vi "Starter Kit FPGA Main.vi"() -> ()   [LabVIEW 2017, in "NI_Robotics_Starter Kit 1.0 FPGA.lvlib"]
doc: "This VI implements the low level control of the motors and sensor for the Starter Kit robot."
uses:
  <vilib>/robotics/Starter Kit/1.0/FPGA Source/NI_Robotics_Starter Kit 1.0 FPGA.lvlib
  <vilib>/Platform/TimedLoop/XDataNode/XDataNode.xnode
  <vilib>/Platform/TimedLoop/XDataNode/nitl_modes.ctl
  <vilib>/Platform/TimedLoop/XDataNode/XDNodeRunTimeDep.lvlib
  <vilib>/Platform/TimedLoop/XDataNode/wakeup.ctl
  <vilib>/Platform/TimedLoop/XDataNode/timing_clust.ctl
  <vilib>/eio/EIONode/EIONode.xnode
  <vilib>/robotics/Utilities/Encoder Count Encoding.ctl
  <vilib>/robotics/Utilities/NI_Robotics Utilities.lvlib
  <vilib>/robotics/Utilities/FPGA Utilities/NI_Robotics_FPGA Utilities.lvlib
  <vilib>/robotics/Utilities/FPGA Utilities/Generate Digital Pulse (uSec).vi
  <vilib>/robotics/Utilities/FPGA Utilities/Count Two Phase Digital Encoder.vi
  <vilib>/robotics/Starter Kit/FPGA Source/NI_Robotics_Starter Kit FPGA.lvlib
  <instrlib>/Parallax Standard Servo/FPGA/NI_Robotics_Parallax Standard Servo (FPGA).lvlib
  <instrlib>/Parallax PING)))/FPGA/NI_Robotics_Parallax PING))) (FPGA).lvlib
  <instrlib>/Sharp IR GP2D12/FPGA/NI_Robotics_Sharp IR GP2D12 (FPGA).lvlib
  <vilib>/addons/control/pid/fpga.llb/XNode/niFpgaPID.xnode
  <vilib>/robotics/Starter Kit/1.0/FPGA Source/Globals.vi
  <vilib>/rvi/eio/common/nirviEmuTemplateMethod_errors.vi
panel:
  in  "FPGA LED":bool
  in  "ModB/AO0":fxp<+/-,20,5> format="%.17g"
  in  "ModB/AO1":fxp<+/-,20,5> format="%.17g"
  in  "ModB/AO2":fxp<+/-,20,5> format="%.17g"
  in  "ModB/AO3":fxp<+/-,20,5> format="%.17g"
  out "ModA/AI0":fxp<+/-,26,5> format="%.23g"
  out "ModA/AI1":fxp<+/-,26,5> format="%.23g"
  out "ModA/AI2":fxp<+/-,26,5> format="%.23g"
  out "ModA/AI3":fxp<+/-,26,5> format="%.23g"
  out "ModA/AI7":fxp<+/-,26,5> format="%.23g"
  out "ModA/AI6":fxp<+/-,26,5> format="%.23g"
  out "ModA/AI5":fxp<+/-,26,5> format="%.23g"
  out "ModA/AI4":fxp<+/-,26,5> format="%.23g"
  out "ModA/AI9":fxp<+/-,26,5> format="%.23g"
  out "ModA/AI8":fxp<+/-,26,5> format="%.23g"
  in  "Port7/DIO0_PWM":T1={"period (us)"=20000, "pulse width (us)"=1500}
  in  "Port7/DIO1_PWM":T1={"period (us)"=20000, "pulse width (us)"=1500}
  in  "Port7/DIO2_PWM":T1={"period (us)"=20000, "pulse width (us)"=1500}
  in  "Port7/DIO3_PWM":T1={"period (us)"=20000, "pulse width (us)"=1500}
  in  "DCmotor_1_direct":bool
  in  "DCmotor_0_direct":bool
  in  "servo_0_direct":bool
  in  "DCmotor_1_PWM":T1={"period (us)"=20000, "pulse width (us)"=1500}
  in  "DCmotor_0_PWM":T1={"period (us)"=20000, "pulse width (us)"=1500}
  in  "servo_0_PWM":T1={"period (us)"=20000, "pulse width (us)"=1500}
  in  "Port3/DIO0":bool
  in  "Port3/DIO0_write":bool
  in  "Port3/DIO1":bool
  in  "Port3/DIO1_write":bool
  in  "Port3/DIO2":bool
  in  "Port3/DIO2_write":bool
  in  "Port3/DIO3":bool
  in  "Port3/DIO3_write":bool
  in  "Port3/DIO4":bool
  in  "Port3/DIO4_write":bool
  in  "Port3/DIO5":bool
  in  "Port3/DIO5_write":bool
  in  "Port3/DIO6":bool
  in  "Port3/DIO6_write":bool
  in  "Port3/DIO7":bool
  in  "Port3/DIO7_write":bool
  in  "Port3/DIO8":bool
  in  "Port3/DIO8_write":bool
  in  "Port3/DIO9":bool
  in  "Port3/DIO9_write":bool
  out "GP2D12_0_voltage":fxp<+/-,26,5> format="%.23g"
  in  "GP2D12_0_calparams":T2={"m"=3.028200149536133, "b"=0.30049991607666016, "k"=0.04309988021850586}
  out "GP2D12_0_dist":fxp<+/-,31,13>
  in  "servo_0_ccw offset":fxp<+/-,32,4>
  in  "servo_0_ccw angle":fxp<+/-,32,4>
  out "PING)))_0_timeout":bool
  out "PING)))_0_dist":fxp<+,32,8> format="%.27g"
  out "DCmotor_1_ccw vel":fxp<+/-,32,11>
  out "DCmotor_0_ccw vel":fxp<+/-,32,11>
  in  "DCmotor_1_ccw vel sp":fxp<+/-,32,11>
  in  "DCmotor_0_ccw vel sp":fxp<+/-,32,11>
  in  "stop":bool
  in  "motor PID gains":T3={"proportional gain (Kc)"=0.25, "integral gain (Kc*Ts/Ti)"=0.3984375, "derivative gain (Kc*Td/Ts)"=0.01171875}
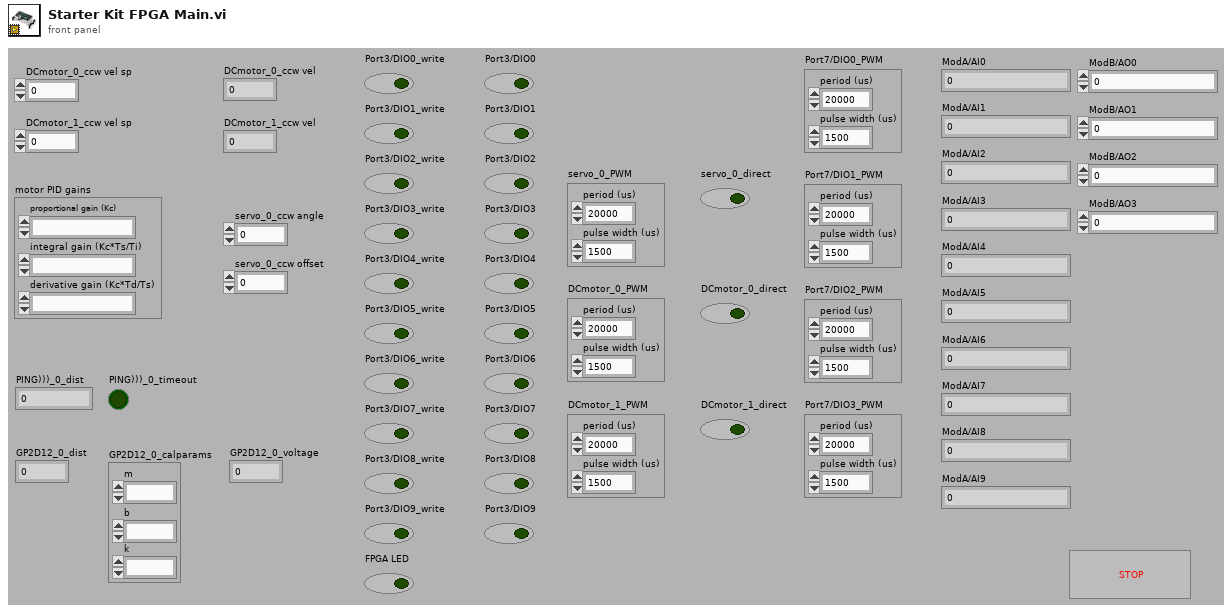
[diagram p1: front panel]
types:
  T1 = cluster{"period (us)":u32, "pulse width (us)":u32}
  T2 = cluster{"m":fxp<+/-,26,5>, "b":fxp<+/-,26,5>, "k":fxp<+/-,26,5>}
  T3 = cluster{"proportional gain (Kc)":fxp<+/-,16,8>, "integral gain (Kc*Ts/Ti)":fxp<+/-,16,8>, "derivative gain (Kc*Td/Ts)":fxp<+/-,16,8>}
  T4 = cluster{"PID gains":cluster{"proportional gain (Kc)":fxp<+/-,16,8>, "integral gain (Kc*Ts/Ti)":fxp<+/-,16,8>, "derivative gain (Kc*Td/Ts)":fxp<+/-,16,8>}, "output range":cluster{"output high":fxp<+/-,16,16>, "output low":fxp<+/-,16,16>}, "setpoint":fxp<+/-,16,16>, "channel index":u16}
  T5 = cluster{"PID gains (x 2^8)":cluster{"proportional gain (Kc)":i16, "integral gain (Kc*Ts/Ti)":i16, "derivative gain (Kc*Td/Ts)":i16}, "output range":cluster{"output high":i16, "output low":i16}, "setpoint":i16, "channel index":u16}
  T6 = typedef "XDNodeRunTimeDep.lvlib/timing_clust.ctl" = cluster{"Expected End [f-1]":u64, "Actual End [f-1]":u64, "Finished Late? [f-1]":bool, "Expected End [i-1]":u64, "Actual End [i-1]":u64, "Finished Late? [i-1]":bool, "Expected Start [i]":u64, "Actual Start [i]":u64, "Expected Start [f]":u64, "Actual Start [f]":u64, "Source Name":string, "Structure Name":string, "Period":i64, "Deadline":i64, "Offset":i64, "Start":i64, "Priority":i32, "Timeout":i32, "Mode":T7, "Wakeup Reason":T8, "Error":errorcluster, "Source Type":string, "Secondary Source Type":string, "Global End Time":u64, "Global Start Time":u64, "Frame Duration":u64, "Iteration Duration":u64, "Assigned CPU":i32, "I/O Scan Engine Mode":u32}
  T7 = typedef "XDNodeRunTimeDep.lvlib/nitl_modes.ctl" = enum32{"No Change", "Process missed periods, maintain original phase", "Discard missed periods, maintain original phase", "Process missed periods, ignore original phase", "Discard missed periods, ignore original phase"}
  T8 = typedef "XDNodeRunTimeDep.lvlib/wakeup.ctl" = enum32{"Normal", "Aborted", "Asynchronous wakeup", "Timing source error", "Timed loop error", "Timeout"}
  T9 = typedef "NI_Robotics Utilities.lvlib/Encoder Count Encoding.ctl" = enum16{"X1", "X2", "X4"}
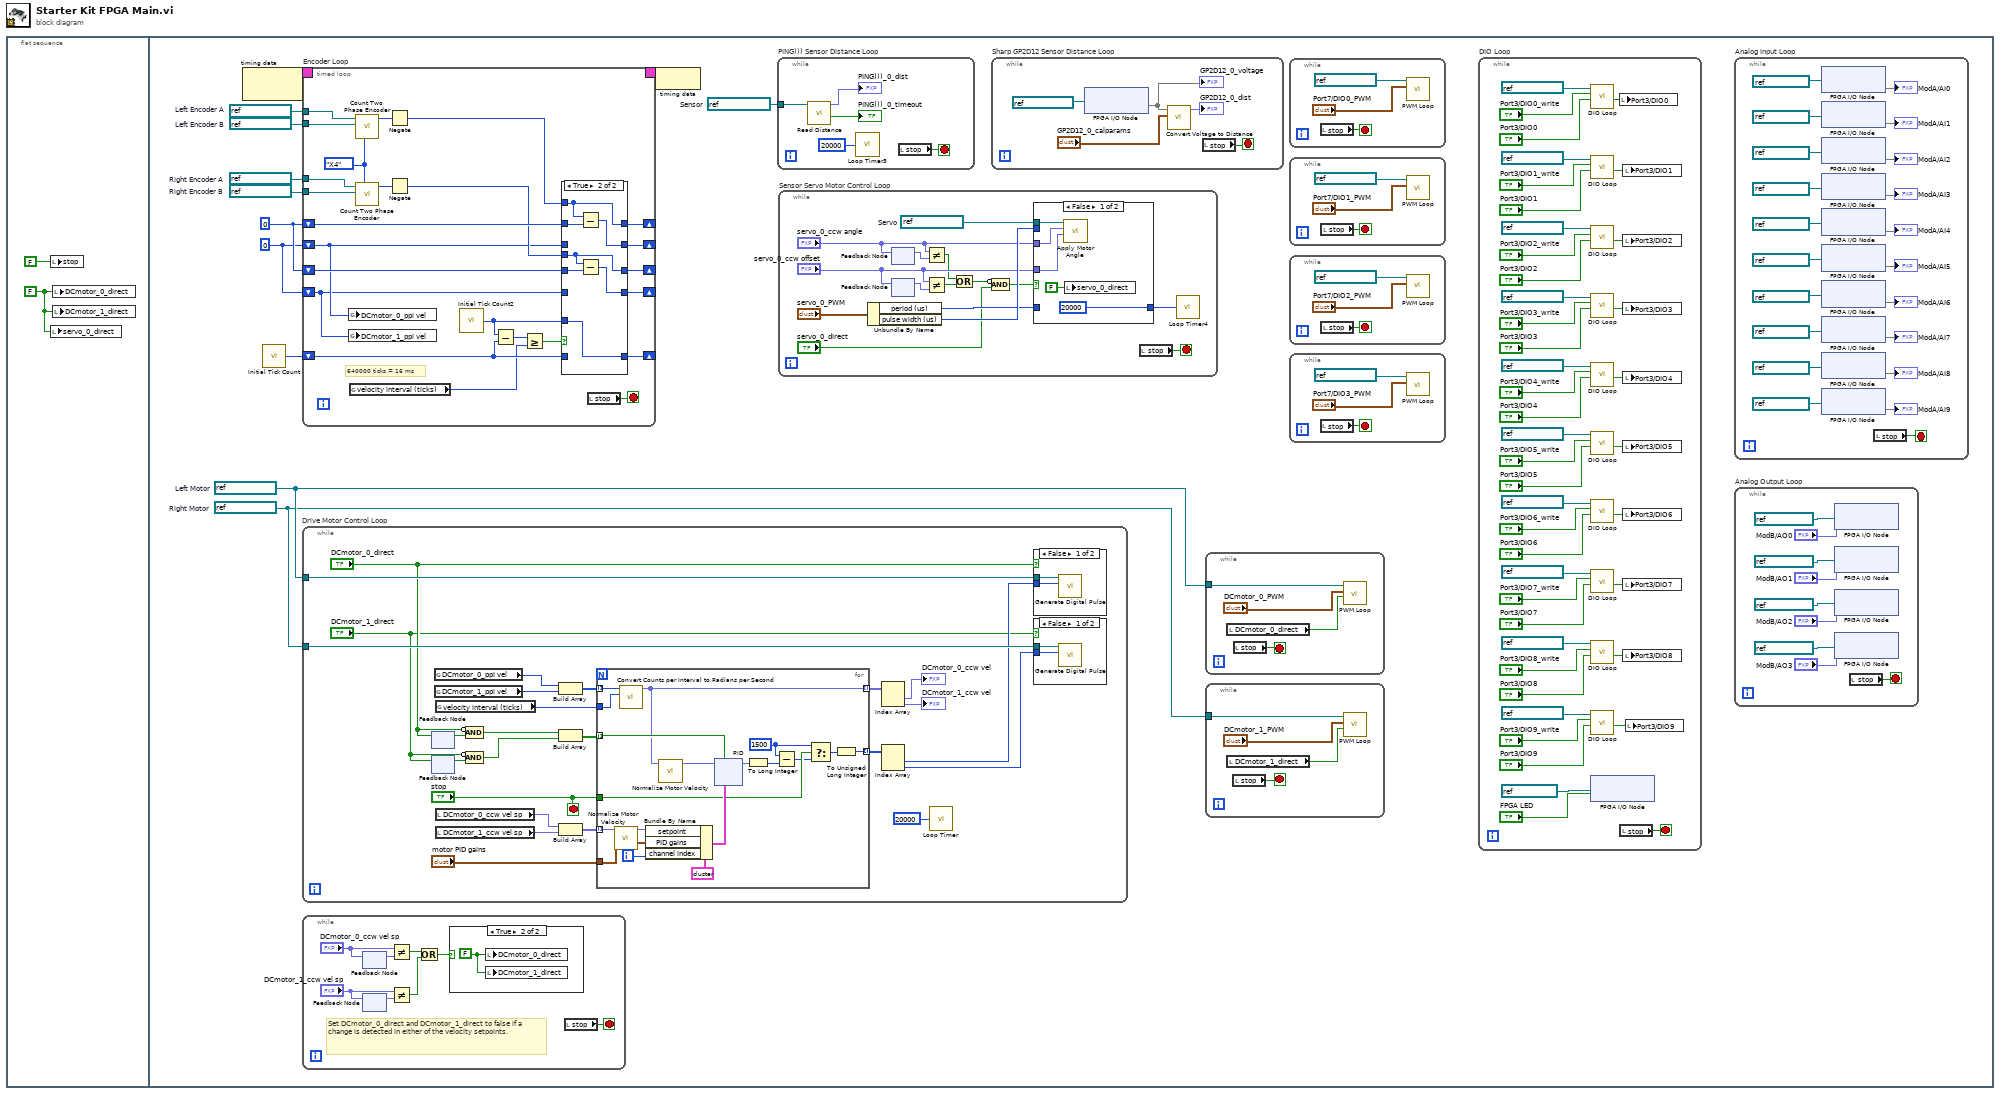
[diagram p0: block diagram]
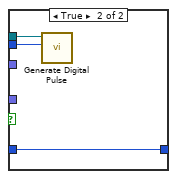
[diagram p3: hidden frame]
diagram:
  n1 = flat-sequence {
    frame #0 {
      w1 = FALSE ("DCmotor_0_direct")
      n2 = local write "stop"(FALSE ("stop")) -> ()
      n3 = local write "servo_0_direct"(w1) -> ()
      n4 = local write "DCmotor_0_direct"(w1) -> ()
      n5 = local write "DCmotor_1_direct"(w1) -> ()
    }
    frame #1 {
      w3 = refnum<k21> "Port0/DIO5"  # Right Motor
      w4 = refnum<k21> "Port0/DIO4"  # Left Motor
      w5 = refnum<k21> "Port0/DIO3"  # Right Encoder B
      w6 = refnum<k21> "Port0/DIO2"  # Right Encoder A
      w7 = refnum<k21> "Port0/DIO1"  # Left Encoder B
      w8 = refnum<k21> "Port0/DIO0"  # Left Encoder A
      w9 = refnum<k21> "Port0/DIO6"  # Sensor
      w10 = 0
      w11 = 0 ("Reset Position Value")
      n6 = node-c288() -> (w14:T6)  [unwired: 1 in]
      n7 = call "Initial Tick Count"() -> ("Tick Count(Ticks)"=w12:u32)
      n8 = while "Drive Motor Control Loop" {
        tunnel: w4 -> [w164]
        tunnel: w3 -> [w166]
        stop <- "stop" stop-if-true
        n9 = feedback #1() -> (w150:bool)  [unwired: 1 in]
        n10 = feedback-in #1("DCmotor_0_direct") -> ()
        n11 = feedback #2() -> (w148:bool)  [unwired: 1 in]
        n12 = feedback-in #2("DCmotor_1_direct") -> ()
        n13 = global read "Globals.vi" "DCmotor_0_ppi vel"() -> (w155:i32)
        n14 = global read "Globals.vi" "DCmotor_1_ppi vel"() -> (w154:i32)
        n15 = global read "Globals.vi" "velocity interval (ticks)"() -> (w153:u32)
        n16 = local read "DCmotor_0_ccw vel sp"() -> (w157:fxp<+/-,32,11>)
        n17 = local read "DCmotor_1_ccw vel sp"() -> (w156:fxp<+/-,32,11>)
        n18 = Compound Arithmetic op=AND(invert "DCmotor_0_direct", w150) -> (w147:bool)
        n19 = Compound Arithmetic op=AND(invert "DCmotor_1_direct", w148) -> (w146:bool)
        n20 = Build Array(w155, w154) -> (w162:i32[])
        n21 = Build Array(w147, w146) -> (w145:bool[])
        n22 = Build Array(w157, w156) -> (w161:fxp<+/-,32,11>[])
        n23 = for {
          tunnel: "motor PID gains" -> [w184]
          tunnel: w162 -> [w179] mode=indexing
          tunnel: w153 -> [w178]
          tunnel: [w177] -> w159 mode=indexing
          tunnel: w161 -> [w174] mode=indexing
          tunnel: "stop" -> [w173]
          tunnel: [w182] -> w158 mode=indexing
          tunnel: w145 -> [w181] mode=indexing
          i -> [w185]
          w172 = 1500 ("y")
          n24 = call <vilib>:"Normalize Motor Velocity.vi"("velocity (rad/s)"=w174) -> ("normalized velocity"=w175:fxp<+/-,16,16>)  [unwired: 10 in]
          n25 = call <vilib>:"Convert Counts per Interval to Radians per Second.vi"("interval (ticks)"=w178, "velocity (pulses/interval)"=w179) -> ("velocity (rad/s)"=w177:fxp<+/-,32,11>)  [unwired: 9 in]
          n26 = Bundle By Name(cluster=T4 {"PID gains"={"proportional gain (Kc)"=0.00390625, "integral gain (Kc*Ts/Ti)"=0.00390625, "derivative gain (Kc*Td/Ts)"=0.00390625}, "output range"={"output high"=500.0, "output low"=-500.0}, "setpoint"=0.0, "channel index"=0} ("configuration"), "setpoint"=w175, "PID gains"=w184, "channel index"=w185) -> (w186:T4)
          n27 = call <vilib>:"Normalize Motor Velocity.vi"("velocity (rad/s)"=w177) -> ("normalized velocity"=w176:fxp<+/-,16,16>)  [unwired: 10 in]
          n28 = xnode ("PID")("process variable"=w176, "reset?"=w181, "configuration"=w186) -> ("output"=w183:fxp<+/-,16,16>)  [unwired: 1 out]
          n29 = To Long Integer(number=w183) -> (32bit integer=w180:i32)
          n30 = Subtract(x=w172, y=w180) -> (x-y=w171:i32)
          n31 = Select(t=w172, s=w173, f=w171) -> (s? t:f=w170:i32)
          n32 = To Unsigned Long Integer(number=w170) -> (unsigned 32bit integer=w182:u32)
        }
        n33 = Index Array(array=w159) -> (element #1=→"DCmotor_0_ccw vel":fxp<+/-,32,11>, element #2=→"DCmotor_1_ccw vel":fxp<+/-,32,11>)  [unwired: 2 in]
        n34 = Index Array(array=w158) -> (element #1=w163:u32, element #2=w165:u32)  [unwired: 2 in]
        n35 = call "Loop Timer"("Count(uSec)"=u32 20000) -> ()  [unwired: 1 out]
        n36 = case shown="False" "DCmotor_0_direct" {
          tunnel: w163 -> [w216 _]
          tunnel: w164 -> [w215 _]
          frame False {
            n37 = call-poly <vilib>:"Generate Digital Pulse.vi"("pulse width (uSec)"=w216, "FPGA digital output"=w215) -> ()  [unwired: 10 in]
          }
          frame True {
          }
        }
        n38 = case shown="False" "DCmotor_1_direct" {
          tunnel: w165 -> [w218 _]
          tunnel: w166 -> [w217 _]
          frame False {
            n39 = call-poly <vilib>:"Generate Digital Pulse.vi"("pulse width (uSec)"=w218, "FPGA digital output"=w217) -> ()  [unwired: 10 in]
          }
          frame True {
          }
        }
      }
      n40 = timed-loop "Encoder Loop" {
        timing: w14 -> [_]
        timing-out: [_] -> w13
        shift-right: [w240] -> _
        shift-left: w12 -> [w245]
        shift-right: [w241] -> _
        shift-left: w11 -> [w243]
        shift-right: [w242] -> _
        shift-left: w10 -> [w227]
        shift-right: [w238] -> _
        shift-left: w11 -> [w239]
        shift-right: [w237] -> _
        shift-left: w10 -> [w226]
        tunnel: w8 -> [w234]
        tunnel: w7 -> [w233]
        tunnel: w6 -> [w231]
        tunnel: w5 -> [w230]
        stop <- w224 stop-if-true
        w228 = Encoder_Count_Encoding."X4" ("count multiplier (X1)")
        # "640000 ticks = 16 ms"
        n41 = global write "Globals.vi" "DCmotor_0_ppi vel"(w227) -> ()
        n42 = global write "Globals.vi" "DCmotor_1_ppi vel"(w226) -> ()
        n43 = global read "Globals.vi" "velocity interval (ticks)"() -> (w225:u32)
        n44 = call-poly <vilib>:"Count Two Phase Encoder.vi"("count encoding (X1)"=w228, "phase B FPGA digital input"=w233, "phase A FPGA digital input"=w234) -> ("new count"=w232:i32)  [unwired: 7 in, 1 out]
        n45 = call-poly <vilib>:"Count Two Phase Encoder.vi"("count encoding (X1)"=w228, "phase B FPGA digital input"=w230, "phase A FPGA digital input"=w231) -> ("new count"=w229:i32)  [unwired: 7 in, 1 out]
        n46 = Negate(x=w232) -> (-x=w236:i32)
        n47 = Negate(x=w229) -> (-x=w235:i32)
        n48 = call "Initial Tick Count2"() -> ("Tick Count(Ticks)"=w244:u32)
        n49 = Subtract(x=w244, y=w245) -> (x-y=w247:u32)
        n50 = Greater Or Equal?(x=w247, y=w225) -> (x >= y?=w246:bool)
        n51 = case shown="True" w246 {
          tunnel: w244 -> [_ w258]
          tunnel: w245 -> [w252 _]
          tunnel: [w252 w258] -> w240
          tunnel: w243 -> [w251 w259]
          tunnel: [w251 w257] -> w241
          tunnel: w236 -> [_ w257]
          tunnel: [w250 w256] -> w242
          tunnel: w227 -> [w250 _]
          tunnel: w239 -> [w249 w255]
          tunnel: w226 -> [w248 _]
          tunnel: [w249 w254] -> w238
          tunnel: [w248 w253] -> w237
          tunnel: w235 -> [_ w254]
          frame False {
          }
          frame True {
            n52 = Subtract(x=w257, y=w259) -> (x-y=w256:i32)
            n53 = Subtract(x=w254, y=w255) -> (x-y=w253:i32)
          }
        }
        n54 = local read "stop"() -> (w224:bool)
      }
      n55 = while {
        stop <- w20 stop-if-true
        # "Set DCmotor_0_direct and DCmotor_1_direct to false if a change is detected in either of the velocity setpoints."
        n56 = feedback-in #3("DCmotor_0_ccw vel sp") -> ()
        n57 = feedback #3() -> (w22:fxp<+/-,32,11>)  [unwired: 1 in]
        n58 = feedback #4() -> (w18:fxp<+/-,32,11>)  [unwired: 1 in]
        n59 = feedback-in #4("DCmotor_1_ccw vel sp") -> ()
        n60 = Not Equal?(x="DCmotor_0_ccw vel sp", y=w22) -> (x != y?=w16:bool)
        n61 = Not Equal?(x="DCmotor_1_ccw vel sp", y=w18) -> (x != y?=w17:bool)
        n62 = Or(x=w16, y=w17) -> (x .or. y?=w15:bool)
        n63 = case shown="True" w15 {
          frame False {
          }
          frame True {
            w23 = FALSE ("DCmotor_0_direct")
            n64 = local write "DCmotor_0_direct"(w23) -> ()
            n65 = local write "DCmotor_1_direct"(w23) -> ()
          }
        }
        n66 = local read "stop"() -> (w20:bool)
      }
      n67 = node-c288(w13) -> ()
      n68 = while "PING))) Sensor Distance Loop" {
        tunnel: w9 -> [w222]
        stop <- w219 stop-if-true
        n69 = call <instrlib>:"Read Distance.vi"("trigger/echo line"=w222) -> ("timed out?"=→"PING)))_0_timeout":bool, "distance (m)"=→"PING)))_0_dist":fxp<+,32,8>)  [unwired: 9 in]
        n70 = call "Loop Timer3"("Count(uSec)"=u32 20000 ("sensor period (15000 us)")) -> ()  [unwired: 1 out]
        n71 = local read "stop"() -> (w219:bool)
      }
      n72 = while "Sensor Servo Motor Control Loop" {
        stop <- w105 stop-if-true
        w118 = refnum<k21> "Port0/DIO7"  # Servo
        n73 = Unbundle By Name("servo_0_PWM") -> ("period (us)"=w115:u32, "pulse width (us)"=w117:u32)
        n74 = feedback-in #5("servo_0_ccw angle") -> ()
        n75 = feedback #5() -> (w114:fxp<+/-,32,4>)  [unwired: 1 in]
        n76 = feedback #6() -> (w111:fxp<+/-,32,4>)  [unwired: 1 in]
        n77 = feedback-in #6("servo_0_ccw offset") -> ()
        n78 = Not Equal?(x="servo_0_ccw angle", y=w114) -> (x != y?=w109:bool)
        n79 = Not Equal?(x="servo_0_ccw offset", y=w111) -> (x != y?=w110:bool)
        n80 = Or(x=w109, y=w110) -> (x .or. y?=w108:bool)
        n81 = Compound Arithmetic op=AND(invert w108, "servo_0_direct") -> (w106:bool)
        n82 = case shown="False" w106 {
          tunnel: w118 -> [w124 w127]
          tunnel: w117 -> [_ w126]
          tunnel: "servo_0_ccw angle" -> [w123 _]
          tunnel: "servo_0_ccw offset" -> [w122 _]
          tunnel: [u32 20000 ("Count(uSec)") w125] -> w116
          tunnel: w115 -> [_ w125]
          frame False {
            n83 = call <instrlib>:"Apply Motor Angle.vi"("ccw angle offset (rad)"=w122, "ccw angle (rad)"=w123, "digital output line"=w124) -> ()  [unwired: 9 in]
            n84 = local write "servo_0_direct"(FALSE ("servo_0_direct")) -> ()
          }
          frame True {
            n85 = call-poly <vilib>:"Generate Digital Pulse.vi"("pulse width (uSec)"=w126, "FPGA digital output"=w127) -> ()  [unwired: 10 in]
          }
        }
        n86 = local read "stop"() -> (w105:bool)
        n87 = call "Loop Timer4"("Count(uSec)"=w116) -> ()  [unwired: 1 out]
      }
      n88 = while "Sharp GP2D12 Sensor Distance Loop" {
        stop <- w128 stop-if-true
        n89 = xnode "FPGA I/O Node"("FPGA I/O In"=refnum<k21> "ModA/AI10") -> ("I/O Item"=w131)  [unwired: 1 out]
        "GP2D12_0_voltage" <- w131
        n90 = call <instrlib>:"Convert Voltage to Distance.vi"("calibration parameters"="GP2D12_0_calparams", "voltage"=w131) -> ("distance (m)"=→"GP2D12_0_dist":fxp<+/-,31,13>)  [unwired: 9 in]
        n91 = local read "stop"() -> (w128:bool)
      }
      n92 = while {
        tunnel: w4 -> [w104]
        stop <- w101 stop-if-true
        n93 = local read "DCmotor_0_direct"() -> (w103:bool)
        n94 = local read "stop"() -> (w101:bool)
        n95 = call <vilib>:"PWM Loop.vi"("generate pulse (T)"=w103, "PWM"="DCmotor_0_PWM", "FPGA I/O"=w104) -> ()  [unwired: 9 in]
      }
      n96 = while {
        tunnel: w3 -> [w100]
        stop <- w97 stop-if-true
        n97 = local read "DCmotor_1_direct"() -> (w99:bool)
        n98 = local read "stop"() -> (w97:bool)
        n99 = call <vilib>:"PWM Loop.vi"("generate pulse (T)"=w99, "PWM"="DCmotor_1_PWM", "FPGA I/O"=w100) -> ()  [unwired: 9 in]
      }
      n100 = while {
        stop <- w142 stop-if-true
        n101 = local read "stop"() -> (w142:bool)
        n102 = call <vilib>:"PWM Loop.vi"("PWM"="Port7/DIO0_PWM", "FPGA I/O"=refnum<k21> "Port7/DIO0" ("FPGA I/O In")) -> ()  [unwired: 10 in]
      }
      n103 = while {
        stop <- w139 stop-if-true
        n104 = local read "stop"() -> (w139:bool)
        n105 = call <vilib>:"PWM Loop.vi"("PWM"="Port7/DIO1_PWM", "FPGA I/O"=refnum<k21> "Port7/DIO1" ("FPGA I/O In")) -> ()  [unwired: 10 in]
      }
      n106 = while {
        stop <- w136 stop-if-true
        n107 = local read "stop"() -> (w136:bool)
        n108 = call <vilib>:"PWM Loop.vi"("PWM"="Port7/DIO2_PWM", "FPGA I/O"=refnum<k21> "Port7/DIO2" ("FPGA I/O In")) -> ()  [unwired: 10 in]
      }
      n109 = while {
        stop <- w133 stop-if-true
        n110 = local read "stop"() -> (w133:bool)
        n111 = call <vilib>:"PWM Loop.vi"("PWM"="Port7/DIO3_PWM", "FPGA I/O"=refnum<k21> "Port7/DIO3" ("FPGA I/O In")) -> ()  [unwired: 10 in]
      }
      n112 = while "DIO Loop" {
        stop <- w54 stop-if-true
        n113 = call <vilib>:"DIO Loop.vi"("DIO value in"="Port3/DIO0", "enable output"="Port3/DIO0_write", "DIO line"=refnum<k21> "Port3/DIO0" ("FPGA I/O")) -> ("DIO value out"=w93:bool)  [unwired: 8 in]
        n114 = call <vilib>:"DIO Loop.vi"("DIO value in"="Port3/DIO1", "enable output"="Port3/DIO1_write", "DIO line"=refnum<k21> "Port3/DIO1" ("FPGA I/O")) -> ("DIO value out"=w92:bool)  [unwired: 8 in]
        n115 = call <vilib>:"DIO Loop.vi"("DIO value in"="Port3/DIO2", "enable output"="Port3/DIO2_write", "DIO line"=refnum<k21> "Port3/DIO2" ("FPGA I/O")) -> ("DIO value out"=w85:bool)  [unwired: 8 in]
        n116 = call <vilib>:"DIO Loop.vi"("DIO value in"="Port3/DIO3", "enable output"="Port3/DIO3_write", "DIO line"=refnum<k21> "Port3/DIO3" ("FPGA I/O")) -> ("DIO value out"=w84:bool)  [unwired: 8 in]
        n117 = call <vilib>:"DIO Loop.vi"("DIO value in"="Port3/DIO4", "enable output"="Port3/DIO4_write", "DIO line"=refnum<k21> "Port3/DIO4" ("FPGA I/O")) -> ("DIO value out"=w77:bool)  [unwired: 8 in]
        n118 = call <vilib>:"DIO Loop.vi"("DIO value in"="Port3/DIO5", "enable output"="Port3/DIO5_write", "DIO line"=refnum<k21> "Port3/DIO5" ("FPGA I/O")) -> ("DIO value out"=w76:bool)  [unwired: 8 in]
        n119 = call <vilib>:"DIO Loop.vi"("DIO value in"="Port3/DIO6", "enable output"="Port3/DIO6_write", "DIO line"=refnum<k21> "Port3/DIO6" ("FPGA I/O")) -> ("DIO value out"=w69:bool)  [unwired: 8 in]
        n120 = call <vilib>:"DIO Loop.vi"("DIO value in"="Port3/DIO7", "enable output"="Port3/DIO7_write", "DIO line"=refnum<k21> "Port3/DIO7" ("FPGA I/O")) -> ("DIO value out"=w68:bool)  [unwired: 8 in]
        n121 = call <vilib>:"DIO Loop.vi"("DIO value in"="Port3/DIO8", "enable output"="Port3/DIO8_write", "DIO line"=refnum<k21> "Port3/DIO8" ("FPGA I/O")) -> ("DIO value out"=w61:bool)  [unwired: 8 in]
        n122 = call <vilib>:"DIO Loop.vi"("DIO value in"="Port3/DIO9", "enable output"="Port3/DIO9_write", "DIO line"=refnum<k21> "Port3/DIO9" ("FPGA I/O")) -> ("DIO value out"=w60:bool)  [unwired: 8 in]
        n123 = xnode "FPGA I/O Node"("I/O Item"="FPGA LED", "FPGA I/O In"=refnum<k21> "FPGA LED" ("LED")) -> ()  [unwired: 1 out]
        n124 = local write "Port3/DIO0"(w93) -> ()
        n125 = local read "stop"() -> (w54:bool)
        n126 = local write "Port3/DIO1"(w92) -> ()
        n127 = local write "Port3/DIO2"(w85) -> ()
        n128 = local write "Port3/DIO3"(w84) -> ()
        n129 = local write "Port3/DIO4"(w77) -> ()
        n130 = local write "Port3/DIO5"(w76) -> ()
        n131 = local write "Port3/DIO6"(w69) -> ()
        n132 = local write "Port3/DIO7"(w68) -> ()
        n133 = local write "Port3/DIO8"(w61) -> ()
        n134 = local write "Port3/DIO9"(w60) -> ()
      }
      n135 = while "Analog Input Loop" {
        stop <- w33 stop-if-true
        n136 = xnode "FPGA I/O Node"("FPGA I/O In"=refnum<k21> "ModA/AI0") -> ("I/O Item"=→"ModA/AI0")  [unwired: 1 out]
        n137 = xnode "FPGA I/O Node"("FPGA I/O In"=refnum<k21> "ModA/AI1") -> ("I/O Item"=→"ModA/AI1")  [unwired: 1 out]
        n138 = xnode "FPGA I/O Node"("FPGA I/O In"=refnum<k21> "ModA/AI2") -> ("I/O Item"=→"ModA/AI2")  [unwired: 1 out]
        n139 = xnode "FPGA I/O Node"("FPGA I/O In"=refnum<k21> "ModA/AI3") -> ("I/O Item"=→"ModA/AI3")  [unwired: 1 out]
        n140 = xnode "FPGA I/O Node"("FPGA I/O In"=refnum<k21> "ModA/AI4") -> ("I/O Item"=→"ModA/AI4")  [unwired: 1 out]
        n141 = xnode "FPGA I/O Node"("FPGA I/O In"=refnum<k21> "ModA/AI5") -> ("I/O Item"=→"ModA/AI5")  [unwired: 1 out]
        n142 = xnode "FPGA I/O Node"("FPGA I/O In"=refnum<k21> "ModA/AI6") -> ("I/O Item"=→"ModA/AI6")  [unwired: 1 out]
        n143 = xnode "FPGA I/O Node"("FPGA I/O In"=refnum<k21> "ModA/AI7") -> ("I/O Item"=→"ModA/AI7")  [unwired: 1 out]
        n144 = xnode "FPGA I/O Node"("FPGA I/O In"=refnum<k21> "ModA/AI8") -> ("I/O Item"=→"ModA/AI8")  [unwired: 1 out]
        n145 = xnode "FPGA I/O Node"("FPGA I/O In"=refnum<k21> "ModA/AI9") -> ("I/O Item"=→"ModA/AI9")  [unwired: 1 out]
        n146 = local read "stop"() -> (w33:bool)
      }
      n147 = while "Analog Output Loop" {
        stop <- w24 stop-if-true
        n148 = xnode "FPGA I/O Node"("I/O Item"="ModB/AO0", "FPGA I/O In"=refnum<k21> "ModB/AO0") -> ()  [unwired: 1 out]
        n149 = xnode "FPGA I/O Node"("I/O Item"="ModB/AO1", "FPGA I/O In"=refnum<k21> "ModB/AO1") -> ()  [unwired: 1 out]
        n150 = xnode "FPGA I/O Node"("I/O Item"="ModB/AO2", "FPGA I/O In"=refnum<k21> "ModB/AO2") -> ()  [unwired: 1 out]
        n151 = xnode "FPGA I/O Node"("I/O Item"="ModB/AO3", "FPGA I/O In"=refnum<k21> "ModB/AO3") -> ()  [unwired: 1 out]
        n152 = local read "stop"() -> (w24:bool)
      }
    }
  }
